vi "FTW-TestExecutive-Launch.vi"(5 "Step Name Dictionary":cluster{"Name":string, "Path":string}[](array[cluster]), 9 "Timeout":i32=-2 format="%d msec", 11 "error in":errorcluster) -> (4 "FTW Actor Connector":refnum<class "FTW-ActorConnector.lvclass">, 6 "Initialized Response":string, 8 "Instance Inbox Address":string, 15 "error out":errorcluster)   [LabVIEW 2015]
uses:
  Connector/FTW-ActorConnector.lvclass
  core/FTW-TestExecutive-Core.lvclass
  container/FTW-Container.lvclass
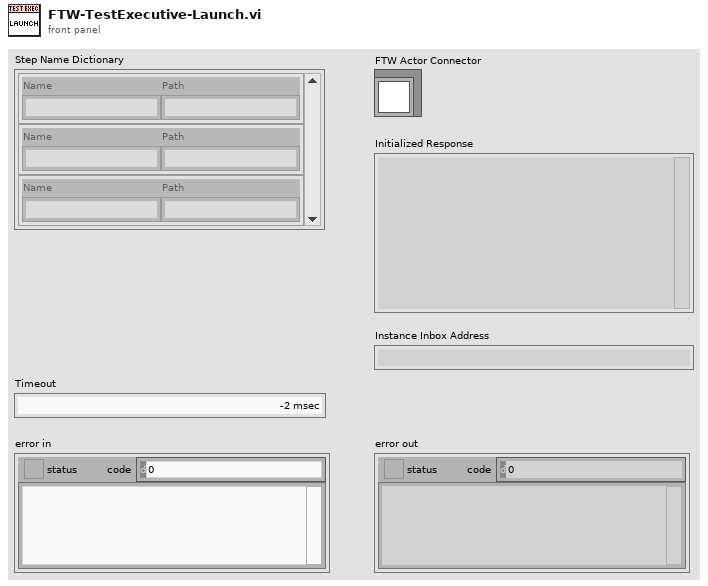
[diagram p1: front panel]
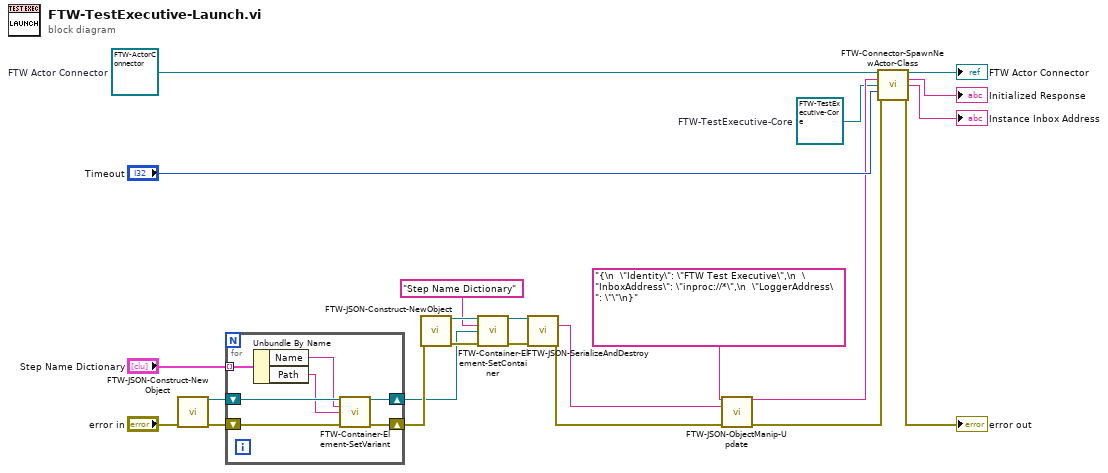
[diagram p0: block diagram]
diagram:
  w14 = refnum<class "FTW-TestExecutive-Core.lvclass"> refnum  # FTW-TestExecutive-Core
  w23 = refnum<class "FTW-ActorConnector.lvclass"> refnum  # FTW Actor Connector
  n1 = call "FTW-JSON-Construct-NewObject.vi"("error in"="error in") -> ("JSON"=w10:refnum<class "FTW-Container.lvclass">, "error out"=w11:errorcluster)  [unwired: 13 in]
  n2 = for {
    tunnel: "Step Name Dictionary" -> [w30] mode=indexing
    shift-right: [w24] -> w9
    shift-left: w11 -> [w28]
    shift-right: [w25] -> w5
    shift-left: w10 -> [w29]
    n3 = Unbundle By Name(w30) -> ("Name"=w27:string, "Path"=w26:string)
    n4 = call "FTW-Container-Element-SetVariant.vi"("FTW-Container In"=w29, "Element Name"=w27, "Variant"=w26, "error in"=w28) -> ("FTW-Container Out"=w25:refnum<class "FTW-Container.lvclass">, "error out"=w24:errorcluster)  [unwired: 9 in, 1 out]
  }
  n5 = call "FTW-JSON-Construct-NewObject.vi"("error in"=w9) -> ("JSON"=w6:refnum<class "FTW-Container.lvclass">, "error out"=w7:errorcluster)  [unwired: 13 in]
  n6 = call "FTW-Container-Element-SetContainer.vi"("FTW-Container In"=w6, "Element Name"="Step Name Dictionary", "Container"=w5, "error in"=w7) -> ("FTW-Container Out"=w2:refnum<class "FTW-Container.lvclass">, "error out"=w8:errorcluster)  [unwired: 9 in, 1 out]
  n7 = call "FTW-JSON-SerializeAndDestroy.vi"("JSON"=w2, "error in"=w8) -> ("JSON String (UTF-8)"=w1:string, "error out"=w3:errorcluster)  [unwired: 12 in]
  n8 = call "FTW-JSON-ObjectManip-Update.vi"("Input JSON Object"="{\n  \"Identity\": \"FTW Test Executive\",\n  \"InboxAddress\": \"inproc://*\",\n  \"LoggerAddress\": \"\"\n}" ("Configuration"), "JSON Object to Merge"=w1, "error in"=w3) -> ("Output JSON Object"=w16:string, "error out"=w15:errorcluster)  [unwired: 11 in]
  n9 = call "FTW-Connector-SpawnNewActor-Class.vi"("FTW Actor Connector Type"=w23, "Configuration"=w16, "Actor Instance"=w14, "Timeout"="Timeout", "error in"=w15) -> ("FTW Actor Connector"=→"FTW Actor Connector":refnum<class "FTW-ActorConnector.lvclass">, "Initialized Response"=→"Initialized Response":string, "Instance Inbox Address"=→"Instance Inbox Address":string, "error out"=→"error out":errorcluster)  [unwired: 7 in]
